vi "Finish.vi"(8 "error in (no error)":errorcluster, 11 "Dev Elevator in":refnum<class "Dev Elevator.lvclass">) -> (0 "error out":errorcluster, 3 "Dev Elevator out":refnum<class "Dev Elevator.lvclass">)   [LabVIEW 2014, in "Dev Elevator.lvlib" / "Dev Elevator.lvclass"]
uses:
  Dev Elevator.lvclass
  Dev Elevator.lvclass/Dev Elevator.ctl
  Robot/Elevator/Elevator Class/Elevator.lvclass
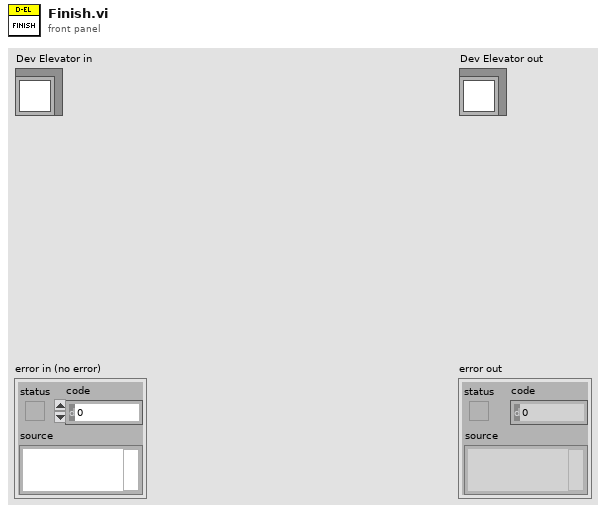
[diagram p1: front panel]
types:
  T1 = typedef "WPI_SolenoidDevRef.ctl" = cluster{"DevStatus":errorcluster, "Pneumatics Control Module":u8, "Forward Solenoid Channel":T2, "Reverse Solenoid Channel":T2}
  T2 = typedef "WPI_SolenoidChannel.ctl" = enum8{"Solenoid 0", "Solenoid 1", "Solenoid 2", "Solenoid 3", "Solenoid 4", "Solenoid 5", "Solenoid 6", "Solenoid 7", "Invalid"}
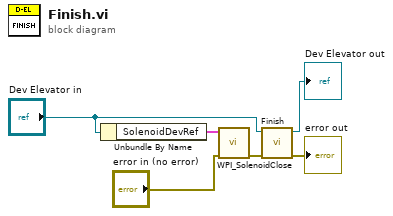
[diagram p0: block diagram]
diagram:
  n1 = Unbundle By Name("Dev Elevator in") -> ("SolenoidDevRef"=w3:T1)
  n2 = call <vilib>:"WPI_SolenoidClose.vi"("error in (no error)"="error in (no error)", "SolenoidDevRef"=w3) -> ("error out"=w1:errorcluster)  [unwired: 9 in]
  n3 = call-parent "Finish.vi"("error in (no error)"=w1, "System Actor in"="Dev Elevator in") -> ("error out"=→"error out":errorcluster, "System Actor out"=→"Dev Elevator out":refnum<class "Dev Elevator.lvclass">)  [unwired: 8 in]
